vi "Plot Helper.vi"   [LabVIEW 2017, in "2D Error Bar Datatype.lvclass"]
doc: "Graphs a plot that displays the percentage or vector of error at each point above and below the line graph. Multiple references to this VI generate multiple plots on the same graph."
uses:
  <vilib>/Math Plots/2D Math Plots/2D Error Bar/2D Error Bar Datatype/2D Error Bar Datatype.lvclass
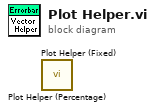
[diagram p0: block diagram]
diagram:
  n1 = call <vilib>:"Plot Helper (Percentage).vi"() -> ()  [unwired: 10 in, 2 out]
  n2 = call <vilib>:"Plot Helper (Fixed).vi"() -> ()  [unwired: 10 in, 2 out]
